vi "Unit_Test.vi"   [LabVIEW 2020]
uses:
  Model/Real Hardware/Stage_MadCityLab/Stage_MadCityLab/Stage_MadCityLab.lvclass
  C:/Program Files/National Instruments/LabVIEW 2020/vi.lib/ActorFramework/Actor/Actor.lvclass
  <vilib>/ActorFramework/Actor/Actor.lvclass
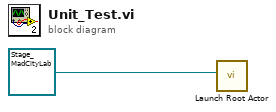
[diagram p0: block diagram]
diagram:
  n1 = call <vilib>:"Launch Root Actor.vi"("Actor"=refnum<class "Stage_MadCityLab.lvclass"> refnum ("Stage_MadCityLab.lvlib:Stage_MadCityLab.lvclass")) -> ()  [unwired: 9 in, 2 out]
